vi "Sharpeness.vi"(0 "Image In (U16)":u16[][](array[numeric]), 11 "Mask Size":dbl) -> (8 "Sharpness":dbl)   [LabVIEW 2016]
uses:
  <vilib>/Analysis/2dsp.llb/2D Real FFT.vi
  <vilib>/Analysis/NI_AALPro.lvlib
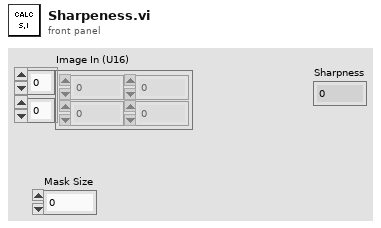
[diagram p1: front panel]
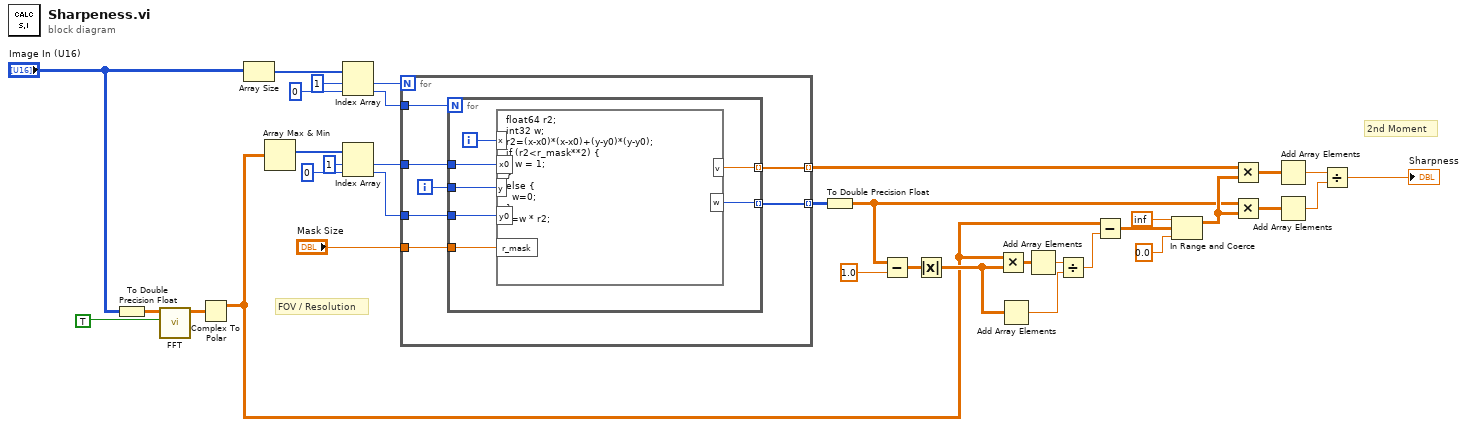
[diagram p0: block diagram]
diagram:
  # "FOV / Resolution"
  # "2nd Moment"
  n1 = To Double Precision Float(number="Image In (U16)") -> (double precision float=w5:dbl[][])
  n2 = call-poly <vilib>:"FFT.vi"("shift?"=TRUE, "X"=w5) -> ("FFT {X}"=w34:cdb[][])  [unwired: 2 in, 7 out]
  n3 = Complex To Polar(r * e^(i*theta)=w34) -> (r=w8:dbl[][])  [unwired: 1 out]
  n4 = Array Size(array="Image In (U16)") -> (size(s)=w20:i32[])
  n5 = Array Max & Min(array=w8) -> (max index (indices)=w33:i32[])  [unwired: 3 out]
  n6 = Index Array(array=w20, index #1=1 ("index"), index #2=0 ("index")) -> (element #1=w17:i32, element #2=w18:i32)
  n7 = Index Array(array=w33, index #1=1 ("index"), index #2=0 ("index")) -> (element #1=w30:i32, element #2=w29:i32)
  n8 = for {
    N: w17 -> [_]
    tunnel: w18 -> [w42]
    tunnel: w30 -> [w41]
    tunnel: w29 -> [w40]
    tunnel: [w39] -> w28 mode=indexing
    tunnel: [w37] -> w4 mode=indexing
    tunnel: "Mask Size" -> [w36]
    i -> [w38]
    n9 = for {
      N: w42 -> [_]
      tunnel: w41 -> [w47]
      tunnel: w40 -> [w45]
      tunnel: [w49] -> w39 mode=indexing
      tunnel: w38 -> [w46]
      tunnel: [w44] -> w37 mode=indexing
      tunnel: w36 -> [w43]
      i -> [w48]
      n10 = formula code="float64 r2;\nint32 w;\nr2=(x-x0)*(x-x0)+(y-y0)*(y-y0);\nif (r2<r_mask**2) {\n   w = 1;\n}\nelse {\n  w=0;\n}\nv=w * r2;"("x"=w48, "x0"=w47, "y"=w46, "y0"=w45, "r_mask"=w43) -> ("v"=w49:dbl, "w"=w44:i32)
    }
  }
  n11 = To Double Precision Float(number=w4) -> (double precision float=w3:dbl[][])
  n12 = Subtract(x=w3, y=1.0) -> (x-y=w14:dbl[][])
  n13 = Absolute Value(x=w14) -> (abs(x)=w9:dbl[][])
  n14 = Multiply(x=w8, y=w9) -> (x*y=w12:dbl[][])
  n15 = Add Array Elements(numeric array=w9) -> (sum=w10:dbl)
  n16 = Add Array Elements(numeric array=w12) -> (sum=w11:dbl)
  n17 = Divide(x=w11, y=w10) -> (x/y=w7:dbl)
  n18 = Subtract(x=w8, y=w7) -> (x-y=w23:dbl[][])
  n19 = In Range and Coerce(upper limit=inf, x=w23, lower limit=0.0) -> (coerced(x)=w13:dbl[][])  [unwired: 1 out]
  n20 = Multiply(x=w28, y=w13) -> (x*y=w27:dbl[][])
  n21 = Multiply(x=w3, y=w13) -> (x*y=w16:dbl[][])
  n22 = Add Array Elements(numeric array=w27) -> (sum=w25:dbl)
  n23 = Add Array Elements(numeric array=w16) -> (sum=w26:dbl)
  n24 = Divide(x=w25, y=w26) -> (x/y=→"Sharpness":dbl)
